vi "zadanie_1.vi"() -> ()   [LabVIEW 2020]
panel:
  out "wyjscie 2":string
  in  "wejscie 2":string
  in  "stop":bool
  out "wyjscie":string
  in  "wejscie":string
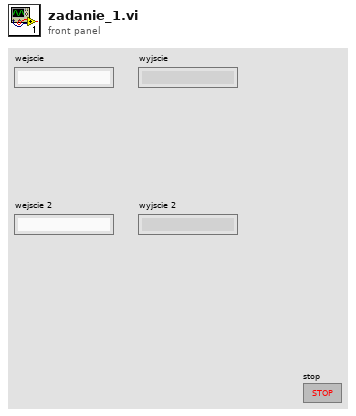
[diagram p1: front panel]
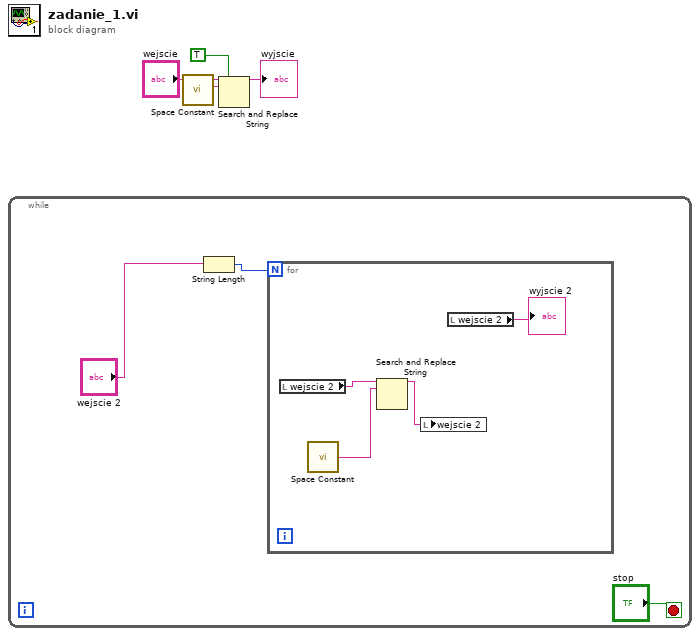
[diagram p0: block diagram]
diagram:
  n1 = while {
    stop <- "stop" stop-if-true
    n2 = String Length(string="wejscie 2") -> (length=w6:i32)
    n3 = for {
      N: w6 -> [_]
      n4 = local read "wejscie 2"() -> (w11:string)
      n5 = call <vilib>:"Space Constant.vi"() -> ("String"=w10:string)
      n6 = Search and Replace String(input string=w11, search string=w10) -> (result string=w8:string)  [unwired: 6 in, 3 out]
      n7 = local write "wejscie 2"(w8) -> ()
      n8 = local read "wejscie 2"() -> (→"wyjscie 2":string)
    }
  }
  n9 = call <vilib>:"Space Constant.vi"() -> ("String"=w2:string)
  n10 = Search and Replace String(replace all?=TRUE ("replace all? (F)"), input string="wejscie", search string=w2) -> (result string=→"wyjscie":string)  [unwired: 5 in, 3 out]
